vi "FPGAmain_5782_phase_PID_v2.vi"() -> ()   [LabVIEW 2013]
uses:
  FPGA/DataMode.ctl
  FPGA/Input_5782/5782_states.ctl
  <vilib>/Platform/TimedLoop/XDataNode/timing_clust.ctl
  <vilib>/Platform/TimedLoop/XDataNode/nitl_modes.ctl
  <vilib>/Platform/TimedLoop/XDataNode/wakeup.ctl
  <vilib>/rvi/Emulation/niFpgaSctlEmulationGetInTimedLoop.vi
  <vilib>/rvi/Emulation/niFpgaEmulationReportErrorSimple.vi
  <vilib>/rvi/Emulation/niFpgaGetClockAttributes.vi
  <vilib>/rvi/Emulation/niFpgaCriticalErrorInLSC.vi
  <vilib>/rvi/DataTransferAndStorage/Register/Emulation/niFpgaRegisterEmulationFpgaImpl.vi
  <instcachedir>/0/niFpgaRegisterEmulationFpgaImpl_DCF4BC0110594B98B44A971D60CEEC4D.lvgen/niFpgaRegisterEmulationFpgaImpl_DCF4BC0110594B98B44A971D60CEEC4D_005.vi
  <vilib>/rvi/DataTransferAndStorage/Container/Common/niFpgaContainerGetUniqueNameForEmu.vi
  <instcachedir>/0/niFpgaRegisterEmulationFpgaImpl_DCF4BC0110594B98B44A971D60CEEC4D.lvgen/niFpgaRegisterEmulationFpgaImpl_DCF4BC0110594B98B44A971D60CEEC4D_014.vi
  <instcachedir>/0/niFpgaRegisterEmulationFpgaImpl_DCF4BC0110594B98B44A971D60CEEC4D.lvgen/niFpgaRegisterEmulationFpgaImpl_DCF4BC0110594B98B44A971D60CEEC4D_013.vi
  <instcachedir>/0/niFpgaRegisterEmulationFpgaImpl_DCF4BC0110594B98B44A971D60CEEC4D.lvgen/niFpgaRegisterEmulationFpgaImpl_DCF4BC0110594B98B44A971D60CEEC4D_011.vi
  <instcachedir>/0/niFpgaRegisterEmulationFpgaImpl_DCF4BC0110594B98B44A971D60CEEC4D.lvgen/niFpgaRegisterEmulationFpgaImpl_DCF4BC0110594B98B44A971D60CEEC4D_010.vi
  <instcachedir>/0/niFpgaRegisterEmulationFpgaImpl_DCF4BC0110594B98B44A971D60CEEC4D.lvgen/niFpgaRegisterEmulationFpgaImpl_DCF4BC0110594B98B44A971D60CEEC4D_015.vi
  <vilib>/rvi/FIFO/Fifo_Resource/nirvififoEmulationReadFpgaImpl.vi
  <vilib>/rvi/interface/RandomDataEmulation/nirviRandomDataMultiElementFPGAFIFO.vi
  <instcachedir>/0/nirviRandomDataMultiElementFPGAFIFO_F2B80EDE0D7944A08478D8D26097D4DB.lvgen/nirviRandomDataMultiElementFPGAFIFO_F2B80EDE0D7944A08478D8D26097D4DB_005.vi
  <vilib>/rvi/interface/RandomDataEmulation/niFpgaRandomDataHandleErrors.vi
  <instcachedir>/0/niFpgaRegisterEmulationFpgaImpl_DCF4BC0110594B98B44A971D60CEEC4D.lvgen/niFpgaRegisterEmulationFpgaImpl_DCF4BC0110594B98B44A971D60CEEC4D_009.vi
  <vilib>/rvi/interface/RandomDataEmulation/nirviRandomDataFPGAFIFO.vi
  <vilib>/rvi/eio/common/nirviEmuTemplateMethod_errors.vi
  <vilib>/rvi/FIFO/Fifo_Resource/nirvififoEmulationWriteFpgaImpl.vi
  <vilib>/Platform/TimedLoop/XDataNode/XDataNode.xnode
  <vilib>/rvi/DataTransferAndStorage/Container/XNode/niFpgaContainer.xnode
  <vilib>/rvi/DataTransferAndStorage/Register/Emulation/niFpgaRegisterEmulation.vi
  <vilib>/rvi/FIFO/Fifo_Resource/nirvififoEmulationRead.vi
  <vilib>/rvi/interface/RandomDataEmulation/nirviRandomDataFpgaMultiElementTemplate.vi
  <vilib>/rvi/interface/RandomDataEmulation/nirviRandomDataFpgaReadWriteTemplate.vi
  <vilib>/eio/EIONode/EIONode.xnode
  <vilib>/rvi/FIFO/Fifo_Resource/nirvififoEmulationWrite.vi
  <vilib>/Platform/TimedLoop/XDataNode/XDNodeRunTimeDep.lvlib
panel:
  in  "new coeffs":bool
  in  "IO Module\\AO Data Sync":bool
  in  "IO Module\\SPI Write Data":u16
  out "IO Module\\SPI Read Data":u8
  in  "IO Module\\SPI Read":bool
  in  "IO Module\\SPI Write":bool
  in  "IO Module\\SPI Address":u16
  in  "IO Module\\SPI Device":u8
  out "IO Module\\SPI Idle":bool
  in  "delay phase":fxp<+,64,64>
  in  "AM phase":fxp<+,64,64>
  in  "User Command Commit":bool
  in  "User Command":u8
  out "User Command Idle":bool
  out "User Command Status":u8
  in  "User Data 0":u8
  in  "User Data 1":u8
  out "PLL Locked":bool
  out "User Error":bool
  out "Configured?":bool
  in  "Continuous":bool
  in  "5782 record length":u16=4000 caption="Samples Per Trigger" min=1 step=1
  in  "Trigger Acquisition":bool
  out "IO Module\\Trigger Input":bool
  in  "Downsample":fxp<+,8,8>=1.0
  in  "FIR coeffs":fxp<+/-,18,18>[](array[numeric])
  in  "CIC Gain":fxp<+/-,32,1>=0.00390625 format="%#_32g"
  in  "Acquisition running":bool
  in  "Phase output":fxp<+,64,64>[](array[numeric])=[0.0, 0.0, 0.0, 0.0, 0.0, 0.0, 0.0, 0.0]
  in  "Simulated phase 5782":fxp<+,64,64>[](array[numeric])=[0.0, 0.0]
  in  "Mode":T1
  in  "Phase 5782":fxp<+,64,64>[](array[numeric])=[0.0, 0.0]
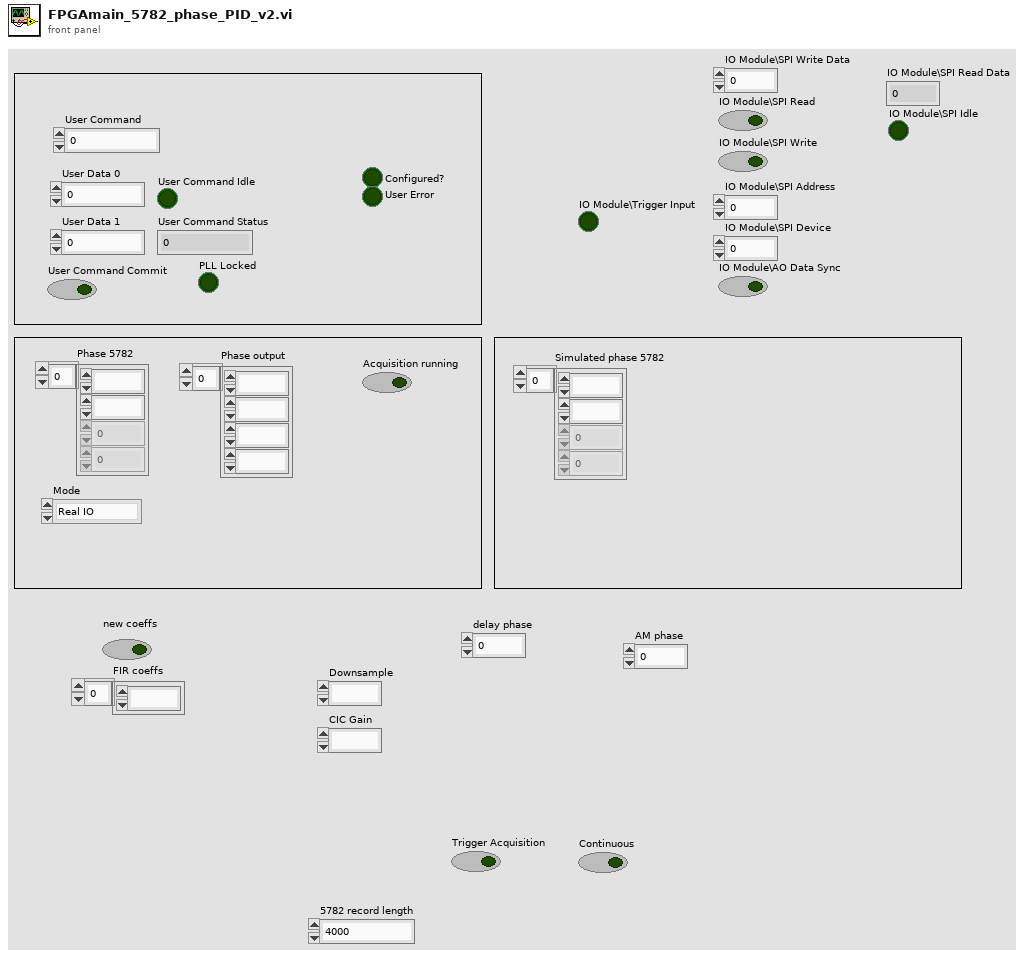
[diagram p1: front panel]
types:
  T1 = typedef "DataMode.ctl" = enum16{"Real IO", "Simulated"}
  T2 = typedef "5782_states.ctl" = enum8{"Wait for trigger", "Acquisition", "Send record length", "Quiet period"}
  T3 = typedef "XDNodeRunTimeDep.lvlib/timing_clust.ctl" = cluster{"Expected End [f-1]":u64, "Actual End [f-1]":u64, "Finished Late? [f-1]":bool, "Expected End [i-1]":u64, "Actual End [i-1]":u64, "Finished Late? [i-1]":bool, "Expected Start [i]":u64, "Actual Start [i]":u64, "Expected Start [f]":u64, "Actual Start [f]":u64, "Source Name":string, "Structure Name":string, "Period":i64, "Deadline":i64, "Offset":i64, "Start":i64, "Priority":i32, "Timeout":i32, "Mode":T4, "Wakeup Reason":T5, "Error":errorcluster, "Source Type":string, "Secondary Source Type":string, "Global End Time":u64, "Global Start Time":u64, "Frame Duration":u64, "Iteration Duration":u64, "Assigned CPU":i32, "I/O Scan Engine Mode":u32}
  T4 = typedef "XDNodeRunTimeDep.lvlib/nitl_modes.ctl" = enum32{"No Change", "Process missed periods, maintain original phase", "Discard missed periods, maintain original phase", "Process missed periods, ignore original phase", "Discard missed periods, ignore original phase"}
  T5 = typedef "XDNodeRunTimeDep.lvlib/wakeup.ctl" = enum32{"Normal", "Aborted", "Asynchronous wakeup", "Timing source error", "Timed loop error", "Timeout"}
  T6 = typedef "I16 array size 2.ctl" = i16[]
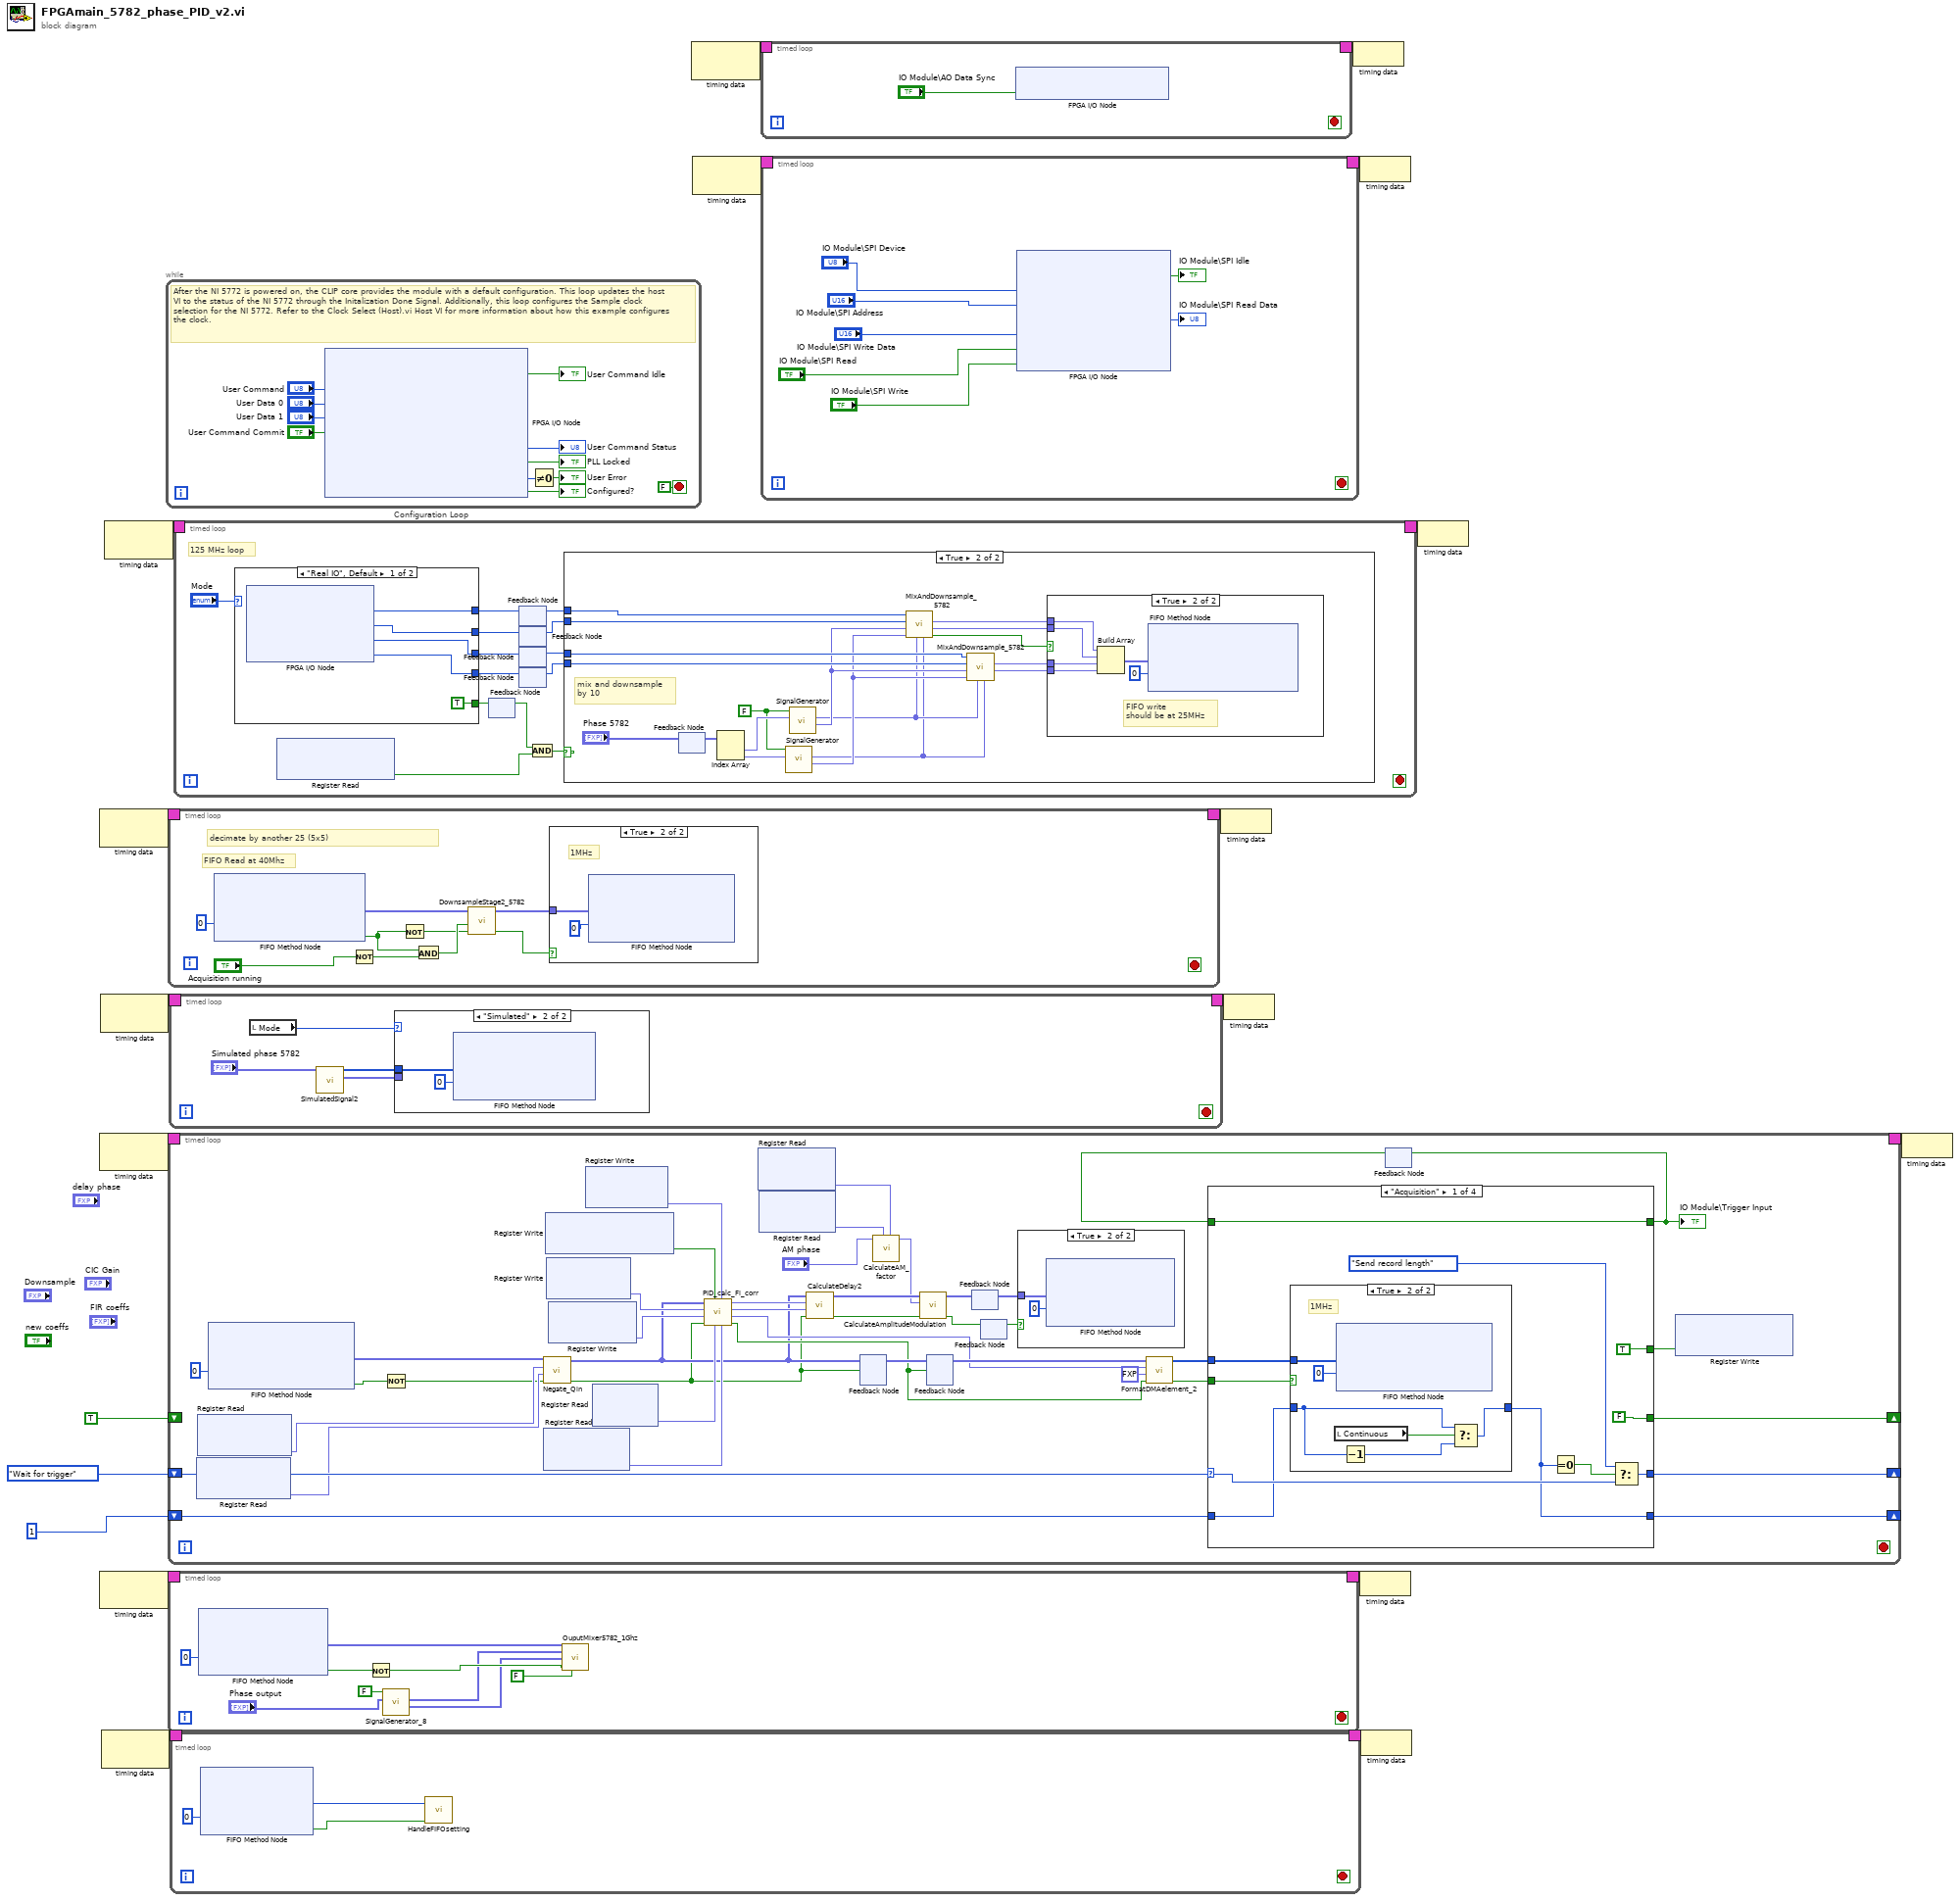
[diagram p0: block diagram]
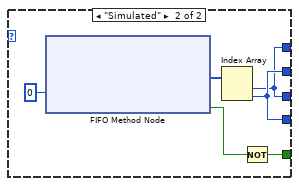
[diagram p4: hidden frame]
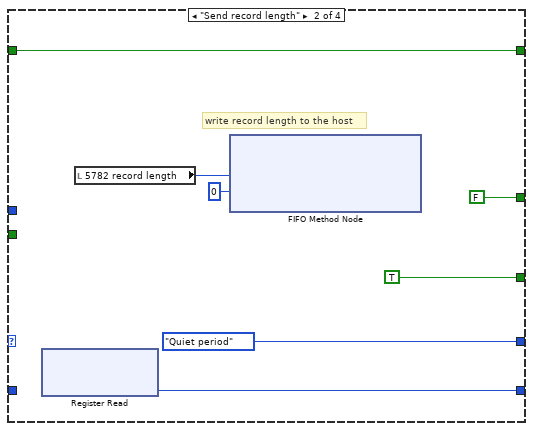
[diagram p7: hidden frame]
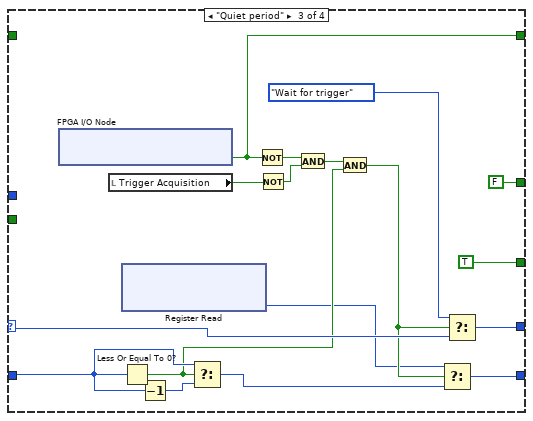
[diagram p8: hidden frame]
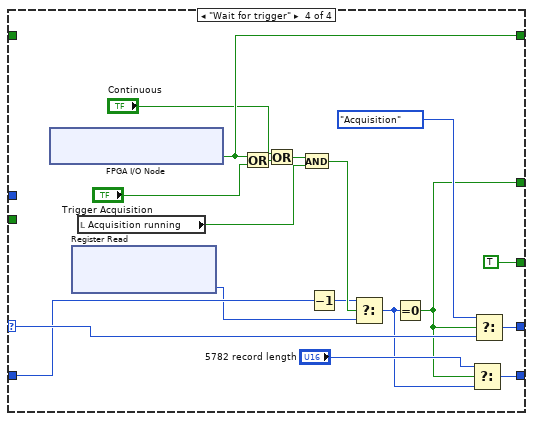
[diagram p9: hidden frame]
diagram:
  n1 = node-c288() -> (w19:T3)  [unwired: 1 in]
  n2 = node-c288() -> (w15:T3)  [unwired: 1 in]
  n3 = node-c288() -> (w10:T3)  [unwired: 1 in]
  n4 = node-c288() -> (w17:T3)  [unwired: 1 in]
  n5 = node-c288() -> (w8:T3)  [unwired: 1 in]
  n6 = node-c288() -> (w2:T3)  [unwired: 1 in]
  n7 = while "Configuration Loop" {
    stop <- FALSE stop-if-true
    # "After the NI 5772 is powered on, the CLIP core provides the module with a default configuration. This loop updates the host VI to the status of the NI 5772 through the Initalization Done Signal. Additionally, this loop configures the Sample clock selection for the NI 5772. Refer to the Clock Select (Host).vi Host VI for more information about how this example configures the clock."
    n8 = xnode "FPGA I/O Node"("IO Module\\User Command"="User Command", "IO Module\\User Data 0"="User Data 0", "IO Module\\User Data 1"="User Data 1", "IO Module\\User Command Commit"="User Command Commit") -> ("IO Module\\User Command Idle"=→"User Command Idle":bool, "IO Module\\User Command Status"=→"User Command Status":u8, "IO Module\\PLL Locked"=→"PLL Locked":bool, "IO Module\\User Error"=w25:u8, "IO Module\\Initialization Done"=→"Configured?":bool)  [unwired: 9 in, 9 out]
    n9 = Not Equal To 0?(x=w25) -> (x != 0?=→"User Error":bool)
  }
  n10 = timed-loop {
    timing: w19 -> [_]
    timing-out: [_] -> w18
    stop <- _ stop-if-true
    # "FIFO Read at 40Mhz"
    # "decimate by another 25 (5x5)"
    n11 = xnode ("FIFO Method Node")("Timeout"=0) -> ("Element"=w38:fxp<+/-,16,14>[], "Timed Out?"=w34:bool)  [unwired: 1 in, 1 out]
    n12 = Not(x="Acquisition running") -> (.not. x?=w35:bool)
    n13 = Not(x=w34) -> (.not. x?=w32:bool)
    n14 = And(x=w34, y=w35) -> (x .and. y?=w33:bool)
    n15 = call "DownsampleStage2_5782.vi"("valid in"=w32, "reset"=w33, "Data in"=w38) -> ("valid out"=w36:bool, "data out"=w37:fxp<+/-,16,14>[])  [unwired: 7 in]
    n16 = case shown="True" w36 {
      tunnel: w37 -> [_ w40]
      frame False {
      }
      frame True {
        # "1MHz"
        n17 = xnode ("FIFO Method Node")("Element"=w40, "Timeout"=0) -> ()  [unwired: 1 in, 2 out]
      }
    }
  }
  n18 = timed-loop {
    timing: w15 -> [_]
    timing-out: [_] -> w14
    shift-right: [w82] -> _
    shift-left: 5782_states."Wait for trigger" ("5782 states") -> [w84]
    shift-right: [w81] -> _
    shift-left: u16 1 ("trigger samples") -> [w83]
    shift-right: [w76] -> _
    shift-left: TRUE -> [_]
    stop <- _ stop-if-true
    n19 = xnode "Register Read"() -> ("Data"=w67:fxp<+/-,16,14>)  [unwired: 1 in, 1 out]
    n20 = xnode "Register Read"() -> ("Data"=w68:fxp<+/-,16,14>)  [unwired: 1 in, 1 out]
    n21 = xnode ("FIFO Method Node")("Timeout"=0) -> ("Element"=w57:fxp<+/-,16,14>[], "Timed Out?"=w79:bool)  [unwired: 1 in, 1 out]
    n22 = Not(x=w79) -> (.not. x?=w56:bool)
    n23 = call "Negate_Qin.vi"("valid in"=w56, "DC offset chan 1"=w67, "DC offset chan 0"=w68, "Data in"=w57) -> ("valid out"=w44:bool, "Data out"=w45:fxp<+/-,16,14>[])  [unwired: 6 in]
    n24 = xnode "Register Read"() -> ("Data"=w62:fxp<+/-,32,4>)  [unwired: 1 in, 1 out]
    n25 = xnode "Register Write"() -> ("Data"=w59:bool)  [unwired: 1 in, 1 out]
    n26 = xnode "Register Write"() -> ("Data"=w60:fxp<+/-,32,4>)  [unwired: 1 in, 1 out]
    n27 = xnode "Register Write"() -> ("Data"=w61:fxp<+/-,32,4>)  [unwired: 1 in, 1 out]
    n28 = xnode "Register Write"() -> ("Data"=w58:fxp<+/-,32,4>)  [unwired: 1 in, 1 out]
    n29 = xnode "Register Read"() -> ("Data"=w63:fxp<+/-,32,4>)  [unwired: 1 in, 1 out]
    n30 = call "PID_calc_Fi_corr.vi"("Kd/Tau"=w62, "Ki*Tau"=w58, "Kp"=w63, "Enabled"=w59, "input valid"=w44, "Fi_delta"=w61, "Fi_start"=w60, "Data in"=w45) -> ("output valid"=w46:bool, "c out"=w48:fxp<+/-,32,4>, "cos_fi_korr"=w69:fxp<+/-,16,2>, "sin fi_korr"=w70:fxp<+/-,16,2>)
    n31 = xnode ("Register Read")() -> ("Data"=w64:fxp<+/-,16,2>)  [unwired: 1 in, 1 out]
    n32 = xnode ("Register Read")() -> ("Data"=w65:fxp<+/-,16,2>)  [unwired: 1 in, 1 out]
    n33 = call "CalculateDelay2.vi"("input valid"=w44, "cos_fi"=w69, "sin fi"=w70, "Data in"=w45) -> ("output valid"=w50:bool, "Data out"=w72:fxp<+/-,16,14>[])  [unwired: 6 in]
    n34 = feedback #1() -> (w51:fxp<+/-,16,14>[])  [unwired: 1 in]
    n35 = feedback-in #1(w45, w44) -> ()
    n36 = call "CalculateAM_factor.vi"("b_am"=w64, "a_am"=w65, "AM phase"="AM phase") -> ("AM_factor"=w71:fxp<+/-,16,2>)  [unwired: 7 in, 1 out]
    n37 = call "CalculateAmplitudeModulation.vi"("input valid"=w50, "AM_factor"=w71, "Data in"=w72) -> ("output valid"=w53:bool, "Data out"=w55:fxp<+/-,16,14>[])  [unwired: 7 in]
    n38 = feedback #2() -> (w49:fxp<+/-,16,14>[])  [unwired: 1 in]
    n39 = feedback-in #2(w51, w46) -> ()
    n40 = feedback-in #3(w55) -> ()
    n41 = feedback #3() -> (w54:fxp<+/-,16,14>[])  [unwired: 1 in]
    n42 = feedback #4() -> (w52:bool)  [unwired: 1 in]
    n43 = feedback-in #4(w53) -> ()
    n44 = case shown="True" w52 {
      tunnel: w54 -> [_ w85]
      frame False {
      }
      frame True {
        n45 = xnode ("FIFO Method Node")("Element"=w85, "Timeout"=0) -> ()  [unwired: 1 in, 2 out]
      }
    }
    n46 = call "FormatDMAelement_2.vi"("valid in"=w46, "c(t) - AM"=fxp<+/-,32,21> 0.0, "c(t) - Phase"=w48, "Data in"=w49) -> ("valid out"=w77:bool, "Element"=w78:u64[])  [unwired: 6 in]
    n47 = feedback #5() -> (w74:bool)  [unwired: 1 in]
    n48 = case shown="\"Acquisition\"" w84 {
      selector: w84 -> [w97 _ w127 w146]
      tunnel: w83 -> [w93 _ w115 w133]
      tunnel: [w96 5782_states."Quiet period" ("5782 states") w126 w145] -> w82
      tunnel: [w90 w105 w128 w144] -> w81
      tunnel: w78 -> [w91 _ _ _]
      tunnel: w77 -> [w92 _ _ _]
      tunnel: [FALSE TRUE TRUE TRUE] -> w76
      tunnel: [TRUE FALSE ("5782 triggered") FALSE ("5782 triggered") w137] -> w75
      tunnel: [w89 w106 w117 w136] -> w73
      tunnel: w74 -> [w89 w106 _ _]
      frame "Acquisition" {
        n49 = case shown="True" w92 {
          tunnel: w91 -> [_ w104]
          tunnel: [w98 w101] -> w90
          tunnel: w93 -> [w98 w99]
          frame False {
          }
          frame True {
            # "1MHz"
            n50 = local read "Continuous"() -> (w102:bool)
            n51 = xnode ("FIFO Method Node")("Element"=w104, "Timeout"=0) -> ()  [unwired: 1 in, 2 out]
            n52 = Decrement(x=w99) -> (x-1=w100:u16)
            n53 = Select(t=w99, s=w102, f=w100) -> (s? t:f=w101:u16)
          }
        }
        n54 = Equal To 0?(x=w90) -> (x = 0?=w94:bool)
        n55 = Select(t=5782_states."Send record length" ("5782 states"), s=w94, f=w97) -> (s? t:f=w96:T2)
      }
      frame "Send record length" {
        # "write record length to the host"
        n56 = xnode ("Register Read")() -> ("Data"=w105:u16)  [unwired: 1 in, 1 out]
        n57 = local read "5782 record length"() -> (w108:u16)
        n58 = xnode ("FIFO Method Node")("Element"=w108, "Timeout"=0) -> ()  [unwired: 1 in, 2 out]
      }
      frame "Quiet period" {
        n59 = xnode "FPGA I/O Node"() -> ("IO Module\\Trigger Input"=w117:bool)  [unwired: 1 in, 1 out]
        n60 = local read "Trigger Acquisition"() -> (w123:bool)
        n61 = xnode ("Register Read")() -> ("Data"=w112:u16)  [unwired: 1 in, 1 out]
        n62 = Less Or Equal To 0?(x=w115) -> (x <= 0?=w114:bool)
        n63 = Decrement(x=w115) -> (x-1=w116:u16)
        n64 = Select(t=w115, s=w114, f=w116) -> (s? t:f=w113:u16)
        n65 = Not(x=w117) -> (.not. x?=w122:bool)
        n66 = Not(x=w123) -> (.not. x?=w121:bool)
        n67 = And(x=w122, y=w121) -> (x .and. y?=w120:bool)
        n68 = And(x=w120, y=w114) -> (x .and. y?=w125:bool)
        n69 = Select(t=w112, s=w125, f=w113) -> (s? t:f=w128:u16)
        n70 = Select(t=5782_states."Wait for trigger" ("5782 states"), s=w125, f=w127) -> (s? t:f=w126:T2)
      }
      frame "Wait for trigger" {
        n71 = xnode "FPGA I/O Node"() -> ("IO Module\\Trigger Input"=w136:bool)  [unwired: 1 in, 1 out]
        n72 = xnode ("Register Read")() -> ("Data"=w129:u16)  [unwired: 1 in, 1 out]
        n73 = local read "Acquisition running"() -> (w138:bool)
        n74 = Or(x=w136, y="Trigger Acquisition") -> (x .or. y?=w132:bool)
        n75 = Or(x="Continuous", y=w132) -> (x .or. y?=w130:bool)
        n76 = And(x=w130, y=w138) -> (x .and. y?=w139:bool)
        n77 = Decrement(x=w133) -> (x-1=w134:u16)
        n78 = Select(t=w134, s=w139, f=w129) -> (s? t:f=w135:u16)
        n79 = Equal To 0?(x=w135) -> (x = 0?=w137:bool)
        n80 = Select(t="5782 record length", s=w137, f=w135) -> (s? t:f=w144:u16)
        n81 = Select(t=5782_states."Acquisition" ("5782 states"), s=w137, f=w146) -> (s? t:f=w145:T2)
      }
    }
    "IO Module\\Trigger Input" <- w73
    n82 = feedback-in #5(w73) -> ()
    n83 = xnode ("Register Write")("Data"=w75) -> ()  [unwired: 1 in, 1 out]
  }
  n84 = timed-loop {
    timing: w10 -> [_]
    timing-out: [_] -> w9
    stop <- _ stop-if-true
    n85 = xnode ("FIFO Method Node")("Timeout"=0) -> ("Element"=w155:fxp<+/-,16,14>[], "Timed Out?"=w156:bool)  [unwired: 1 in, 1 out]
    n86 = Not(x=w156) -> (.not. x?=w153:bool)
    n87 = call "SignalGenerator_8.vi"("Phase"="Phase output", "reset"=FALSE) -> ("Sine out"=w149:fxp<+/-,16,0>[], "Cosine out"=w150:fxp<+/-,16,0>[])  [unwired: 8 in]
    n88 = call "OuputMixer5782_1Ghz.vi"("reset"=FALSE, "valid in"=w153, "Sine in"=w149, "Cosine in"=w150, "Data in"=w155) -> ()  [unwired: 5 in, 2 out]
  }
  n89 = timed-loop {
    timing: w17 -> [_]
    timing-out: [_] -> w16
    stop <- _ stop-if-true
    n90 = local read "Mode"() -> (w163:T1)
    n91 = call "SimulatedSignal2.vi"("Phase"="Simulated phase 5782") -> ("dummy do not use"=w160:fxp<+/-,16,0>[], "output"=w162:T6)  [unwired: 9 in]
    n92 = case shown="\"Simulated\"" w163 {
      tunnel: w162 -> [_ w164]
      tunnel: w160 -> [_ _]
      frame "Real IO", Default {
      }
      frame "Simulated" {
        n93 = xnode ("FIFO Method Node")("Element"=w164, "Timeout"=0) -> ()  [unwired: 1 in, 2 out]
      }
    }
  }
  n94 = timed-loop {
    timing: w8 -> [_]
    timing-out: [_] -> w7
    stop <- _ stop-if-true
    n95 = xnode ("FIFO Method Node")("Timeout"=0) -> ("Element"=w169:u64, "Timed Out?"=w168:bool)  [unwired: 1 in, 1 out]
    n96 = call "HandleFIFOsetting.vi"("timed out"=w168, "Value"=w169) -> ()  [unwired: 10 in]
  }
  n97 = timed-loop {
    timing: w2 -> [_]
    timing-out: [_] -> w1
    stop <- _ stop-if-true
    # "125 MHz loop"
    n98 = case shown="\"Real IO\", Default" "Mode" {
      tunnel: [w214 w217] -> w184
      tunnel: [w213 w218] -> w182
      tunnel: [w212 w217] -> w180
      tunnel: [w211 w218] -> w177
      tunnel: [TRUE w215] -> w176
      frame "Real IO", Default {
        n99 = xnode "FPGA I/O Node"() -> ("IO Module\\AI 0 N-1"=w214:i16, "IO Module\\AI 0 N"=w213:i16, "IO Module\\AI 1 N-1"=w212:i16, "IO Module\\AI 1 N"=w211:i16)  [unwired: 4 in, 4 out]
      }
      frame "Simulated" {
        n100 = xnode ("FIFO Method Node")("Timeout"=0) -> ("Element"=w219:i16[], "Timed Out?"=w216:bool)  [unwired: 1 in, 1 out]
        n101 = Index Array(array=w219) -> (element #1=w217:i16, element #2=w218:i16)  [unwired: 2 in]
        n102 = Not(x=w216) -> (.not. x?=w215:bool)
      }
    }
    n103 = xnode ("Register Read")() -> ("Data"=w174:bool)  [unwired: 1 in, 1 out]
    n104 = feedback #6() -> (w175:bool)  [unwired: 1 in]
    n105 = feedback-in #6(w176) -> ()
    n106 = feedback #7() -> (w183:i16)  [unwired: 1 in]
    n107 = feedback-in #7(w184) -> ()
    n108 = feedback #8() -> (w181:i16)  [unwired: 1 in]
    n109 = feedback-in #8(w182) -> ()
    n110 = feedback #9() -> (w179:i16)  [unwired: 1 in]
    n111 = feedback-in #9(w180) -> ()
    n112 = feedback #10() -> (w178:i16)  [unwired: 1 in]
    n113 = feedback-in #10(w177) -> ()
    n114 = And(x=w175, y=w174) -> (x .and. y?=w185:bool)
    n115 = case shown="True" w185 {
      tunnel: w183 -> [_ w194]
      tunnel: w181 -> [_ w193]
      tunnel: w179 -> [_ w192]
      tunnel: w178 -> [_ w191]
      frame False {
      }
      frame True {
        w195 = FALSE
        # "mix and downsample\nby 10"
        n116 = feedback #11() -> (w197:fxp<+,64,64>[])  [unwired: 1 in]
        n117 = feedback-in #11("Phase 5782") -> ()
        n118 = Index Array(array=w197) -> (element #1=w196:fxp<+,64,64>, element #2=w198:fxp<+,64,64>)  [unwired: 2 in]
        n119 = call "SignalGenerator.vi"("phase"=w198, "Reset"=w195) -> ("Cos"=w189:fxp<+/-,16,0>, "Sin"=w187:fxp<+/-,16,0>)  [unwired: 7 in, 1 out]
        n120 = call "SignalGenerator.vi"("phase"=w196, "Reset"=w195) -> ("Cos"=w190:fxp<+/-,16,0>, "Sin"=w188:fxp<+/-,16,0>)  [unwired: 7 in, 1 out]
        n121 = call "MixAndDownsample_5782.vi"("sin1"=w187, "sin0"=w188, "cos1"=w189, "cos0"=w190, "signal 1"=w193, "signal 0"=w194) -> ("data valid"=w201:bool, "Q out"=w202:fxp<+/-,16,14>, "I out"=w203:fxp<+/-,16,14>)  [unwired: 3 in]
        n122 = call "MixAndDownsample_5782.vi"("sin1"=w187, "sin0"=w188, "cos1"=w189, "cos0"=w190, "signal 1"=w191, "signal 0"=w192) -> ("Q out"=w199:fxp<+/-,16,14>, "I out"=w200:fxp<+/-,16,14>)  [unwired: 3 in, 1 out]
        n123 = case shown="True" w201 {
          tunnel: w202 -> [_ w209]
          tunnel: w203 -> [_ w206]
          tunnel: w200 -> [_ w205]
          tunnel: w199 -> [_ w204]
          frame False {
          }
          frame True {
            # "FIFO write\nshould be at 25MHz"
            n124 = Build Array(w206, w209, w205, w204) -> (w208:fxp<+/-,16,14>[])
            n125 = xnode ("FIFO Method Node")("Element"=w208, "Timeout"=0) -> ()  [unwired: 1 in, 2 out]
          }
        }
      }
    }
  }
  n126 = node-c288() -> (w4:T3)  [unwired: 1 in]
  n127 = node-c288() -> (w6:T3)  [unwired: 1 in]
  n128 = timed-loop {
    timing: w4 -> [_]
    timing-out: [_] -> w3
    stop <- _ stop-if-true
    n129 = xnode "FPGA I/O Node"("IO Module\\AO Data Sync"="IO Module\\AO Data Sync") -> ()  [unwired: 1 in, 1 out]
  }
  n130 = timed-loop {
    timing: w6 -> [_]
    timing-out: [_] -> w5
    stop <- _ stop-if-true
    n131 = xnode "FPGA I/O Node"("IO Module\\SPI Device"="IO Module\\SPI Device", "IO Module\\SPI Address"="IO Module\\SPI Address", "IO Module\\SPI Write Data"="IO Module\\SPI Write Data", "IO Module\\SPI Read"="IO Module\\SPI Read", "IO Module\\SPI Write"="IO Module\\SPI Write") -> ("IO Module\\SPI Idle"=→"IO Module\\SPI Idle":bool, "IO Module\\SPI Read Data"=→"IO Module\\SPI Read Data":u8)  [unwired: 7 in, 7 out]
  }
  n132 = node-c288(w18) -> ()
  n133 = node-c288(w16) -> ()
  n134 = node-c288(w3) -> ()
  n135 = node-c288(w5) -> ()
  n136 = node-c288(w9) -> ()
  n137 = node-c288(w7) -> ()
  n138 = node-c288(w1) -> ()
  n139 = node-c288(w14) -> ()
